vi "MCL Sort test 2.vi"() -> ()   [LabVIEW 2010]
panel:
  out "STOP (Shots MC LB)":bool=TRUE
  in  "MC Listbox of Shots":i32(listbox)
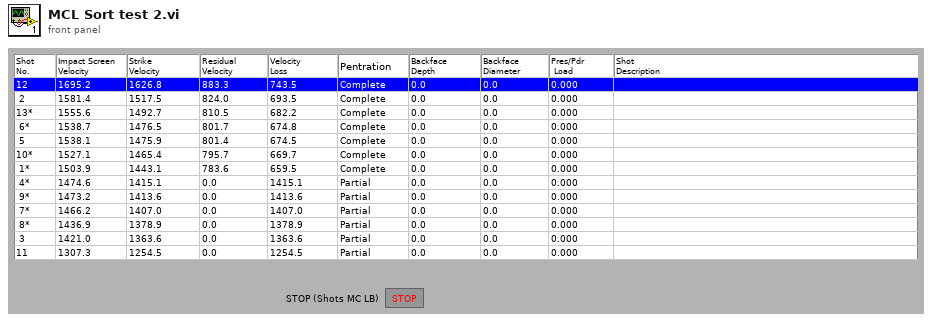
[diagram p1: front panel]
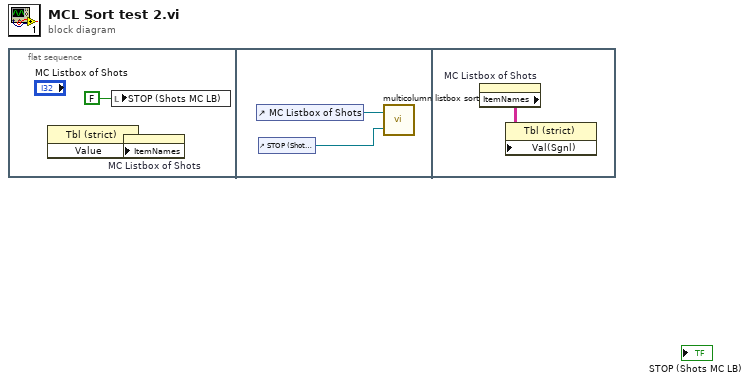
[diagram p0: block diagram]
diagram:
  n1 = flat-sequence {
    frame #0 {
      n2 = property on="Property Node" class="Tbl (strict)"() -> ("Value"=w2:string[][])  [unwired: 2 in, 2 out]
      n3 = local write "STOP (Shots MC LB)"(FALSE ("STOP (Shots MC LB)")) -> ()
      n4 = property on="MC Listbox of Shots" class="MCListbox (strict)"("ItemNames"=w2) -> ()  [unwired: 2 in, 2 out]
    }
    frame #1 {
      n5 = control-ref of="MC Listbox of Shots"() -> (w4:refnum<vi>)
      n6 = control-ref of="STOP (Shots MC LB)"() -> (w3:refnum<vi>)
      n7 = call "multicolumn listbox sort.vi"("Bool Refnum"=w3, "MCListbox Refnum"=w4) -> ()  [unwired: 1 out]
    }
    frame #2 {
      n8 = property on="MC Listbox of Shots" class="MCListbox (strict)"() -> ("ItemNames"=w5:string[][])  [unwired: 2 in, 2 out]
      n9 = property on="Property Node" class="Tbl (strict)"("Val(Sgnl)"=w5) -> ()  [unwired: 2 in, 2 out]
    }
  }
